vi "Field Draw Target.vi"(4 "Lado":enum16{"Esquerdo", "Direito"}(ring) caption="Enum", 6 "Draw Targets?":T2, 7 "Robot":refnum<class "Robot.lvclass">, 8 "picture in":picture, 9 "Offset":T4, 10 "Scale mm/pixel":dbl, 11 "Project":T1=enum."VSS") -> (0 "picture out":picture)   [LabVIEW 2023]
uses:
  <vilib>/Utility/miscctls.llb/LVBoundsTypeDef.ctl
  <vilib>/Analysis/coordinate.llb/Angle Range (Degree).ctl
  DrawTargets.ctl
  Robot_class/Robot.lvclass
  Parameters_class/Project.ctl
  Controls/Functions Enum.ctl
  Robot_class/Robot.lvclass/Robot.ctl
  <vilib>/Analysis/coordinate.llb/2D Cartesian Coordinate Rotation (Scalar).vi
  Robot_class/Read dest_orientation.vi
  Robot_class/Read dest_x.vi
  Robot_class/Read dest_y.vi
  Robot_class/Read dest_x_kick.vi
  Robot_class/Read dest_y_kick.vi
  Robot_class/Read role.vi
  Robot_class/Read tactic.vi
  <vilib>/Analysis/NI_AAL_Angle.lvlib
  <vilib>/Analysis/NI_AALPro.lvlib
  <vilib>/Analysis/coordinate.llb/Wrap Angle (scalar).vi
panel:
  in  "angle range":T3=1
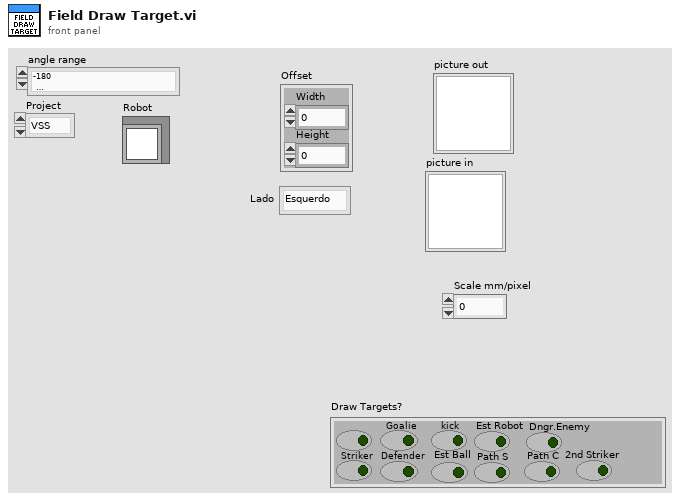
[diagram p1: front panel]
types:
  T1 = typedef "Project.ctl" = enum16{"SSL", "VSS"}
  T2 = typedef "DrawTargets.ctl" = cluster{"Attacker":bool, "Striker":bool, "Goalie":bool, "Defender":bool, "kick":bool, "Est Ball":bool, "Est Robot":bool, "Path S":bool, "Path C":bool, "Dngr.Enemy":bool, "2nd Striker":bool}
  T3 = typedef "NI_AAL_Angle.lvlib/Angle Range (Degree).ctl" = u16
  T4 = typedef "LVBoundsTypeDef.ctl" = cluster{"Width":u32, "Height":u32}
  T5 = typedef "Functions Enum.ctl" = enum16{"2nd Striker", "Attacker", "Goalie", "Defender", "Striker", "Goto 0", "Dummy", "Kicker", "ZigZag 0", "ZigZag 1", "ZigZag 2", "ZigZag 3", "ZigZag 4", "ZigZag 5", "ZigZag 6", "ZigZag 7", "ZigZag 8", ""}
  T6 = typedef "roles.ctl" = enum16{"BallChallengerAttackerVSS", "NormalAttackerVSS", "AttackerAimGoalVSS", "DefenderAreaVSS", "KeeperVSS", "Tabler", "TableFinalizer", "PrepareRollToPassRoller", "PrepareRollToPassReceiver", "SimplePassRoll", "SimplePassRollReceiver", "PenaltyDefense", "PreparePassReceiver 2", "PreparePassReceiver 1", "PassObserver", "Timeout", "Goto", "ZigZag", "None", "BallOutOfField", "DefenderArea", "Duelist", "AttackerStop", "FollowAttacker", "KeeperRole", "KickPenalty", "AttackerAimGoal", "AttackerBlock", "Marker", "Halt", "Shoot", "PassKicker", "PassReceiver", "TestRole", "PenaltyAttacker"}
  T7 = typedef "tactics.ctl" = enum16{"ReceivePassInFuturePoint", "Roller", "PrepareRollToPassRollerGoTo", "PrepareRollToPassReceiverGoTo", "WaitRoll", "PositionToRoll", "PenaltyAttacker", "PassObserver", "PenaltyDefense", "TableReceiverTactic", "Test", "DefendGoal", "Marker", "FollowAttacker", "DefendArea", "Shoot", "AttackerAimGoal", "AttackerBallOutOfField", "AttackerBlock", "AttackerStop", "Duelist", "Halt", "ZigZag", "GoTo", "Timeout", "KickToPassReceiver", "PositionToReceivePass", "DefendAreaVSS", "DefendGoalVSS", "KickVSS", "AttackVSS", "DispBallVSS", "PenaltyAttackVSS", "WaitPass"}
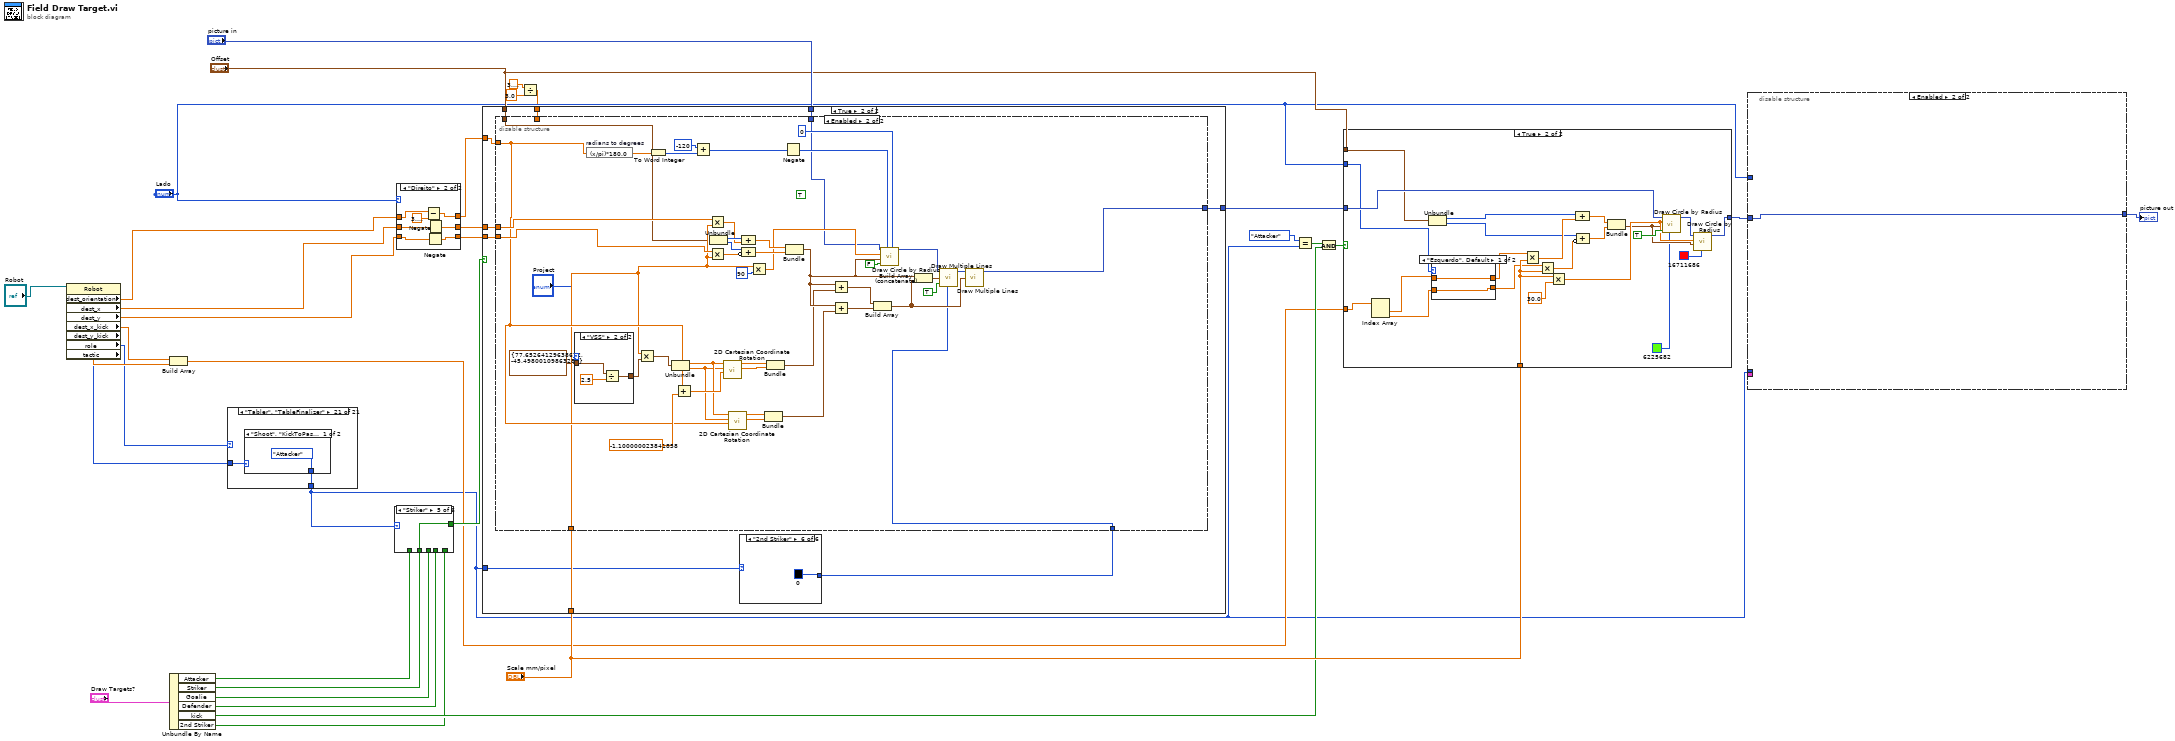
[diagram p0: block diagram]
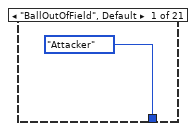
[diagram p2: hidden frame]
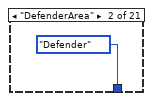
[diagram p3: hidden frame]
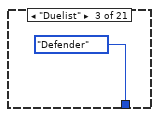
[diagram p4: hidden frame]
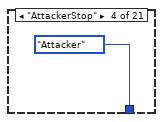
[diagram p5: hidden frame]
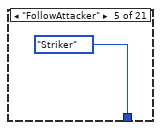
[diagram p6: hidden frame]
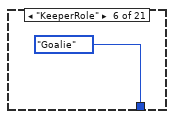
[diagram p7: hidden frame]
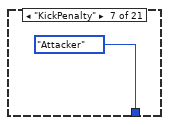
[diagram p8: hidden frame]
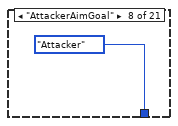
[diagram p9: hidden frame]
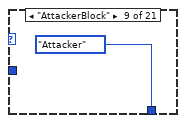
[diagram p10: hidden frame]
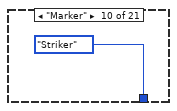
[diagram p11: hidden frame]
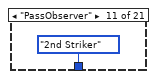
[diagram p12: hidden frame]
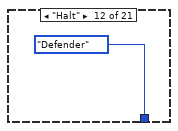
[diagram p13: hidden frame]
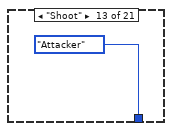
[diagram p14: hidden frame]
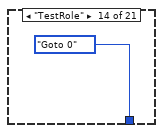
[diagram p15: hidden frame]
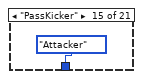
[diagram p16: hidden frame]
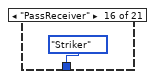
[diagram p17: hidden frame]
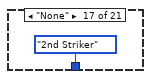
[diagram p18: hidden frame]
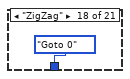
[diagram p19: hidden frame]
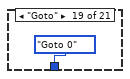
[diagram p20: hidden frame]
diagram:
  n1 = property class="Robot"(reference="Robot") -> ("dest_orientation"=w9:dbl, "dest_x"=w8:dbl, "dest_y"=w7:dbl, "dest_x_kick"=w6:dbl, "dest_y_kick"=w5:dbl, "role"=w3:T6, "tactic"=w1:T7)  [unwired: 1 in, 2 out]
  n2 = Unbundle By Name("Draw Targets?") -> ("Attacker"=w27:bool, "Striker"=w28:bool, "Goalie"=w26:bool, "Defender"=w29:bool, "kick"=w24:bool, "2nd Striker"=w11:bool)
  n3 = Build Array(w6, w5) -> (w4:dbl[])
  n4 = case shown="\"Tabler\", \"TableFinalizer\"" w3 {
    tunnel: [Functions_Enum."Attacker" ("function") Functions_Enum."Defender" ("function") Functions_Enum."Defender" ("function") Functions_Enum."Attacker" ("function") Functions_Enum."Striker" ("function") Functions_Enum."Goalie" ("function") Functions_Enum."Attacker" ("function") Functions_Enum."Attacker" ("function") Functions_Enum."Attacker" ("function") Functions_Enum."Striker" ("function") Functions_Enum."2nd Striker" ("function") Functions_Enum."Defender" ("function") Functions_Enum."Attacker" ("function") Functions_Enum."Goto 0" ("function") Functions_Enum."Attacker" ("function") Functions_Enum."Striker" ("function") Functions_Enum."2nd Striker" ("function") Functions_Enum."Goto 0" ("function") Functions_Enum."Goto 0" ("function") Functions_Enum."Goto 0" ("function") w56] -> w2
    tunnel: w1 -> [_ _ _ _ _ _ _ _ _ _ _ _ _ _ _ _ _ _ _ _ w55]
    frame "BallOutOfField", Default {
    }
    frame "DefenderArea" {
    }
    frame "Duelist" {
    }
    frame "AttackerStop" {
    }
    frame "FollowAttacker" {
    }
    frame "KeeperRole" {
    }
    frame "KickPenalty" {
    }
    frame "AttackerAimGoal" {
    }
    frame "AttackerBlock" {
    }
    frame "Marker" {
    }
    frame "PassObserver" {
    }
    frame "Halt" {
    }
    frame "Shoot" {
    }
    frame "TestRole" {
    }
    frame "PassKicker" {
    }
    frame "PassReceiver" {
    }
    frame "None" {
    }
    frame "ZigZag" {
    }
    frame "Goto" {
    }
    frame "Timeout" {
    }
    frame "Tabler", "TableFinalizer" {
      n5 = case shown="\"Shoot\", \"KickToPassReceiver\"" w55 {
        tunnel: [Functions_Enum."Attacker" ("function") Functions_Enum."Striker" ("function")] -> w56
        frame "Shoot", "KickToPassReceiver" {
        }
        frame "WaitPass", Default {
        }
      }
    }
  }
  n6 = case shown="\"Striker\"" w2 {
    tunnel: [w59 w60 TRUE ("Draw Target Striker?") w62 w63 w64] -> w30
    tunnel: w29 -> [_ _ _ w62 _ _]
    tunnel: w28 -> [_ _ _ _ w63 _]
    tunnel: w27 -> [w59 _ _ _ _ _]
    tunnel: w26 -> [_ w60 _ _ _ _]
    tunnel: w11 -> [_ _ _ _ _ w64]
    frame "Attacker", Default {
    }
    frame "Goalie" {
    }
    frame "Goto 0", "Kicker" {
    }
    frame "Defender" {
    }
    frame "Striker" {
    }
    frame "2nd Striker" {
    }
  }
  n7 = case shown="\"Direito\"" "Lado" {
    tunnel: [w67 w74] -> w21
    tunnel: w8 -> [w67 w71]
    tunnel: [w66 w72] -> w20
    tunnel: w7 -> [w66 w73]
    tunnel: w9 -> [w65 w69]
    tunnel: [w65 w70] -> w16
    frame "Esquerdo", Default {
    }
    frame "Direito" {
      n8 = Subtract(x=w69, y=3.141592653589793) -> (x-y=w70:dbl)
      n9 = Negate(x=w73) -> (-x=w72:dbl)
      n10 = Negate(x=w71) -> (-x=w74:dbl)
    }
  }
  n11 = Divide(x=3.141592653589793, y=3.0) -> (x/y=w15:dbl)
  n12 = case shown="True" w30 {
    tunnel: w20 -> [_ w84]
    tunnel: w21 -> [_ w83]
    tunnel: "picture in" -> [w75 w82]
    tunnel: [w75 w81] -> w33
    tunnel: "Offset" -> [_ w80]
    tunnel: "Scale mm/pixel" -> [_ w79]
    tunnel: w2 -> [_ w78]
    tunnel: w16 -> [_ w77]
    tunnel: w15 -> [_ w76]
    frame False {
    }
    frame True {
      n13 = case shown="\"2nd Striker\"" w78 {
        tunnel: [u32 14047743 ("color(black)") u32 16711680 ("color(black)") u32 11760127 ("color(black)") u32 4390883 ("color(black)") u32 16774186 ("color(black)") u32 0 ("color(black)")] -> w85
        frame "Goalie" {
        }
        frame "Attacker", Default {
        }
        frame "Goto 0", "Kicker" {
        }
        frame "Defender" {
        }
        frame "Striker" {
        }
        frame "2nd Striker" {
        }
      }
      n14 = disable-structure shown="Enabled" {
        disable-tunnel: w85 -> [w123 w129]
        disable-tunnel: w84 -> [w121 w134]
        disable-tunnel: w83 -> [w120 w135]
        disable-tunnel: w82 -> [w113 w132]
        disable-tunnel: [w109 w131] -> w81
        disable-tunnel: w80 -> [w108 w128]
        disable-tunnel: w79 -> [w107 w130]
        disable-tunnel: w77 -> [w98 w133]
        disable-tunnel: w76 -> [w95 _]
        frame Disabled {
          (unwired) 0.0 ("y")
          n15 = Unbundle(w108) -> ("Width"=w119:u32, "Height"=w116:u32)
          n16 = Divide(x=w95, y=2.0) -> (x/y=w97:dbl)
          n17 = Subtract(x=w98, y=w97) -> (x-y=w104:dbl)
          n18 = Multiply(x=w120, y=w107) -> (x*y=w118:dbl)
          n19 = Negate(x=w104) -> (-x=w103:dbl)
          n20 = Multiply(x=w121, y=w107) -> (x*y=w115:dbl)
          n21 = Divide(x=3.141592653589793, y=1.0) -> (x/y=w86:dbl)
          n22 = Multiply(x=w107, y=sgl 50.0 ("radius")) -> (x*y=w111:dbl)
          n23 = Subtract(x=w103, y=w86) -> (x-y=w99:dbl)
          n24 = Compound Arithmetic op=ADD(w119, w118) -> (w117:dbl)
          n25 = Compound Arithmetic op=ADD(w116, invert w115) -> (w114:dbl)
          n26 = call-poly <vilib>:"Wrap Angle.vi"("angle range"="angle range", "angle in"=w99) -> ("angle out"=w96:dbl)  [unwired: 8 in, 1 out]
          n27 = Bundle(w117, w114) -> (w110:cluster{dbl, dbl})  [unwired: 1 in]
          n28 = Multiply(x=w96, y=180.0) -> (x*y=w93:dbl)
          n29 = Divide(x=w93, y=3.141592653589793) -> (x/y=w88:dbl)
          n30 = Multiply(x=w95, y=180.0) -> (x*y=w94:dbl)
          n31 = Divide(x=w94, y=3.141592653589793) -> (x/y=w87:dbl)
          n32 = call <vilib>:"Draw Circle by Radius.vi"("arc size(360)"=w87, "color(black)"=w123, "start angle(0)"=w88, "fill?(F)"=TRUE, "pixel center"=w110, "radius"=w111, "picture"=w113) -> ("new picture"=w112:picture)  [unwired: 4 in]
          n33 = call <vilib>:"Draw Circle by Radius.vi"("arc size(360)"=w87, "color(black)"=u32 16777215, "start angle(0)"=w88, "pixel center"=w110, "radius"=w111, "picture"=w112) -> ("new picture"=w109:picture)  [unwired: 5 in]
        }
        frame Enabled {
          (unwired) TRUE ("fill?(F)")
          n34 = case shown="\"VSS\"" "Project" {
            tunnel: cluster{sgl, sgl} {77.65264, -45.498} ("appended array") -> [w170 w173]
            tunnel: [w170 w171] -> w126
            frame "SSL", Default {
            }
            frame "VSS" {
              n35 = Divide(x=w173, y=2.5) -> (x/y=w171:cluster{dbl, dbl})
            }
          }
          n36 = expression code="(x/pi)*180.0" "radians to degrees"(w133) -> (w161:dbl)
          n37 = Multiply(x=w130, y=w126) -> (x*y=w141:cluster{dbl, dbl})
          n38 = To Word Integer(number=w161) -> (16bit integer=w160:i16)
          n39 = Unbundle(w141) -> (w145:dbl, w144:dbl)
          n40 = Add(x=w133, y=sgl -1.1 ("theta")) -> (x+y=w146:dbl)
          n41 = Add(x=i16 -120, y=w160) -> (x+y=w159:i16)
          n42 = Multiply(x=w135, y=w130) -> (x*y=w167:dbl)
          n43 = Multiply(x=w134, y=w130) -> (x*y=w164:dbl)
          n44 = Unbundle(w128) -> ("Width"=w168:u32, "Height"=w165:u32)
          n45 = call-poly <vilib>:"2D Cartesian Coordinate Rotation.vi"("theta"=w146, "y"=w144, "x"=w145) -> ("y out"=w148:dbl, "x out"=w149:dbl)  [unwired: 6 in, 1 out]
          n46 = call-poly <vilib>:"2D Cartesian Coordinate Rotation.vi"("theta"=w133, "y"=w144, "x"=w145) -> ("y out"=w142:dbl, "x out"=w143:dbl)  [unwired: 6 in, 1 out]
          n47 = Compound Arithmetic op=ADD(w168, w167) -> (w166:dbl)
          n48 = Compound Arithmetic op=ADD(w165, invert w164) -> (w163:dbl)
          n49 = Multiply(x=w130, y=i16 90 ("radius")) -> (x*y=w155:dbl)
          n50 = Bundle("x out"=w143, "y out"=w142) -> (w140:cluster{"x out":dbl, "y out":dbl})  [unwired: 1 in]
          n51 = Bundle("x out"=w149, "y out"=w148) -> (w139:cluster{"x out":dbl, "y out":dbl})  [unwired: 1 in]
          n52 = Negate(x=w159) -> (-x=w157:i16)
          n53 = Bundle(w166, w163) -> (w154:cluster{dbl, dbl})  [unwired: 1 in]
          n54 = Add(x=w154, y=w139) -> (x+y=w137:cluster{dbl, dbl})
          n55 = Add(x=w154, y=w140) -> (x+y=w138:cluster{dbl, dbl})
          n56 = Build Array(w137, w138) -> (w153:cluster{dbl, dbl}[])
          n57 = call <vilib>:"Draw Circle by Radius.vi"("arc size(360)"=i16 0, "start angle(0)"=w157, "fill?(F)"=FALSE, "pixel center"=w154, "radius"=w155, "picture"=w132) -> ("new picture"=w136:picture)  [unwired: 5 in]
          n58 = Build Array (concatenate)(w154, w153) -> (w151:cluster{dbl, dbl}[])
          n59 = call <vilib>:"Draw Multiple Lines.vi"("picture"=w136, "line endpoints"=w151, "fill?(F)"=TRUE, "color(black)"=w129) -> ("new picture"=w152:picture)  [unwired: 5 in]
          n60 = call <vilib>:"Draw Multiple Lines.vi"("picture"=w152, "line endpoints"=w153) -> ("new picture"=w131:picture)  [unwired: 7 in]
        }
      }
    }
  }
  n61 = Equal?(x=Functions_Enum."Attacker" ("y"), y=w2) -> (x = y?=w23:bool)
  n62 = And(x=w23, y=w24) -> (x .and. y?=w25:bool)
  n63 = case shown="True" w25 {
    tunnel: w33 -> [w180 w192]
    tunnel: [w180 w191] -> w19
    tunnel: "Offset" -> [_ w190]
    tunnel: "Scale mm/pixel" -> [_ w189]
    tunnel: "Lado" -> [_ w184]
    tunnel: w4 -> [_ w183]
    frame False {
    }
    frame True {
      n64 = Index Array(array=w183) -> (element #1=w182:dbl, element #2=w181:dbl)  [unwired: 2 in]
      n65 = Unbundle(w190) -> ("Width"=w201:u32, "Height"=w198:u32)
      n66 = case shown="\"Esquerdo\", Default" w184 {
        tunnel: [w205 w209] -> w186
        tunnel: w182 -> [w205 w207]
        tunnel: [w204 w208] -> w185
        tunnel: w181 -> [w204 w206]
        frame "Esquerdo", Default {
        }
        frame "Direito" {
          n67 = Negate(x=w206) -> (-x=w208:dbl)
          n68 = Negate(x=w207) -> (-x=w209:dbl)
        }
      }
      n69 = Multiply(x=w186, y=w189) -> (x*y=w200:dbl)
      n70 = Multiply(x=w185, y=w189) -> (x*y=w197:dbl)
      n71 = Multiply(x=w189, y=sgl 30.0 ("radius")) -> (x*y=w194:dbl)
      n72 = Compound Arithmetic op=ADD(w201, w200) -> (w199:dbl)
      n73 = Compound Arithmetic op=ADD(w198, invert w197) -> (w196:dbl)
      n74 = Bundle(w199, w196) -> (w193:cluster{dbl, dbl})  [unwired: 1 in]
      n75 = call <vilib>:"Draw Circle by Radius.vi"("color(black)"=u32 6225682, "fill?(F)"=TRUE, "pixel center"=w193, "radius"=w194, "picture"=w192) -> ("new picture"=w195:picture)  [unwired: 6 in]
      n76 = call <vilib>:"Draw Circle by Radius.vi"("color(black)"=u32 16711686, "pixel center"=w193, "radius"=w194, "picture"=w195) -> ("new picture"=w191:picture)  [unwired: 7 in]
    }
  }
  n77 = disable-structure shown="Enabled" {
    disable-tunnel: w19 -> [w219 w239]
    disable-tunnel: w2 -> [w218 _]
    disable-tunnel: [w212 w239] -> w18
    disable-tunnel: _ -> [w211 _]
    disable-tunnel: "Lado" -> [w210 _]
    frame Disabled {
      n78 = Equal?(x=Functions_Enum."Striker", y=w218) -> (x = y?=w213:bool)
      n79 = Equal?(x=Functions_Enum."Attacker", y=w218) -> (x = y?=w214:bool)
      n80 = Or(x=w214, y=w213) -> (x .or. y?=w215:bool)
      n81 = case shown="True" w215 {
        tunnel: w219 -> [w220 w228]
        tunnel: [w220 w229] -> w212
        tunnel: w211 -> [_ w232]
        tunnel: w210 -> [_ w222]
        frame False {
        }
        frame True {
          n82 = Unbundle By Name(w232) -> ("Gap Coord"=w230)
          n83 = Index Array(array=w230) -> (element #1=w225, element #2=w224)  [unwired: 2 in]
          n84 = case shown="\"Esquerdo\", Default" w222 {
            tunnel: [w234 w238] -> _
            tunnel: w225 -> [w234 w236]
            tunnel: [w233 w237] -> w223
            tunnel: w224 -> [w233 w235]
            frame "Esquerdo", Default {
            }
            frame "Direito" {
              n85 = Negate(x=w235) -> (-x=w237:dbl)
              n86 = Negate(x=w236) -> (-x=w238:dbl)
            }
          }
          n87 = Bundle By Name(cluster=cluster{"x":i16, "y":i16} {"x"=0, "y"=0} ("end point"), "x"=i16 -4500, "y"=w223) -> (w227:cluster{"x":i16, "y":i16})
          n88 = call <vilib>:"Draw Line.vi"("picture"=w228, "end point"=w227, "color(black)"=u32 6618880) -> ("new picture"=w229:picture)  [unwired: 6 in]
        }
      }
    }
    frame Enabled {
    }
  }
  "picture out" <- w18
